vi "ULx Read (Counter U32 1Chan 1Samp).vi"(0 "task in":refnum<k24>, 9 "timeout":dbl=10.0, 11 "error in":errorcluster) -> (4 "task out":refnum<k24>, 6 "data":u32, 15 "error out":errorcluster)   [LabVIEW 2020]
doc: "Reads a single 32-bit unsigned integer sample from a task that contains a single counter input channel."
uses:
  C:/Users/William/Documents/LV 2020 builds/LeaktestDAQ/Source-v33/ULx_LV.dll
  ULx_LV.dll
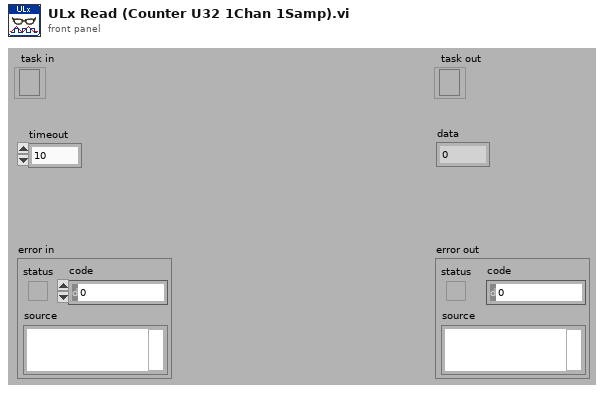
[diagram p1: front panel]
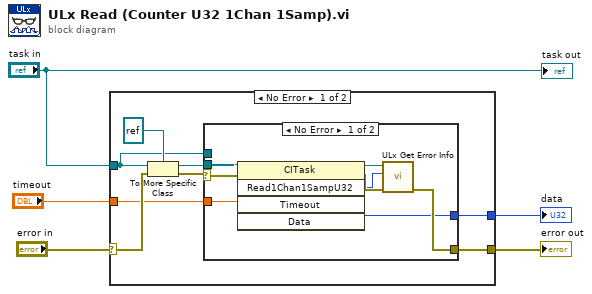
[diagram p0: block diagram]
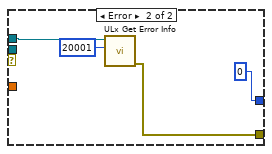
[diagram p2: hidden frame]
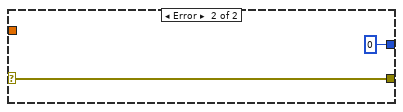
[diagram p3: hidden frame]
diagram:
  n1 = case shown="No Error" "error in" {
    selector: "error in" -> [w13 w27]
    tunnel: "task in" -> [w7 _]
    tunnel: "timeout" -> [w9 _]
    tunnel: [w8 w27] -> w3
    tunnel: [w6 u32 0 ("Read1Chan1SampF64")] -> w1
    frame No Error {
      n2 = To More Specific Class(target class=refnum<k24> refnum, reference=w7, error in=w13) -> (specific class reference=w10:refnum<k24>, error out=w11:errorcluster)
      n3 = case shown="No Error" w11 {
        selector: w11 -> [w20 _]
        tunnel: w10 -> [w21 _]
        tunnel: w9 -> [w19 _]
        tunnel: [w16 w23] -> w8
        tunnel: w7 -> [_ w25]
        tunnel: [w14 u32 0 ("Read1Chan1SampF64")] -> w6
        frame No Error {
          n4 = invoke class="CITask" method="Read1Chan1SampU32"(reference=w21, error in=w20, "Timeout"=w19) -> (reference out=w17:refnum<k24>, error out=w18:errorcluster, "Read1Chan1SampU32"=w15:i32, "Data"=w14:u32)  [unwired: 2 in, 1 out]
          n5 = call "ULx Get Error Info.vi"("error in"=w18, "ErrorCode"=w15, "task in"=w17) -> ("error out"=w16:errorcluster)  [unwired: 8 in]
        }
        frame Error {
          n6 = call "ULx Get Error Info.vi"("ErrorCode"=20001, "task in"=w25) -> ("error out"=w23:errorcluster)  [unwired: 9 in]
        }
      }
    }
    frame Error {
    }
  }
  "data" <- w1
  "error out" <- w3
  "task out" <- "task in"
